vi "AllocateNewError.vi"(8 "ErrorIn":errorcluster, 10 "ErrorCode":i32, 11 "ConnectionIn":refnum<class "Connection.lvclass">) -> (0 "ErrorOut":errorcluster, 3 "ConnectionOut":refnum<class "Connection.lvclass">)   [LabVIEW 2021, in "ErrorDefinitionSQLite.lvclass"]
uses:
  ErrorDefinitionSQLite.lvclass
  ErrorDefinitionSQLite.lvclass/ErrorDefinitionSQLite.ctl
  <vilib>/drjdpowell/SQLite Library/SQLite.lvlib
  <vilib>/drjdpowell/SQLite Library/SQL Connection/Execute SQL.vi
  <vilib>/drjdpowell/SQLite Library/SQL Connection/Connection.lvclass
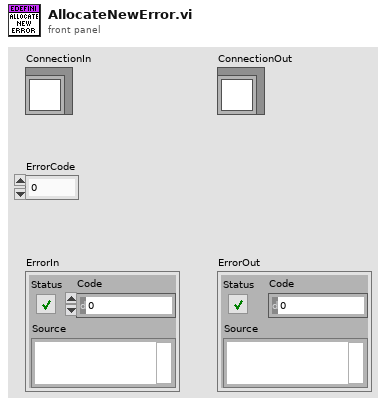
[diagram p1: front panel]
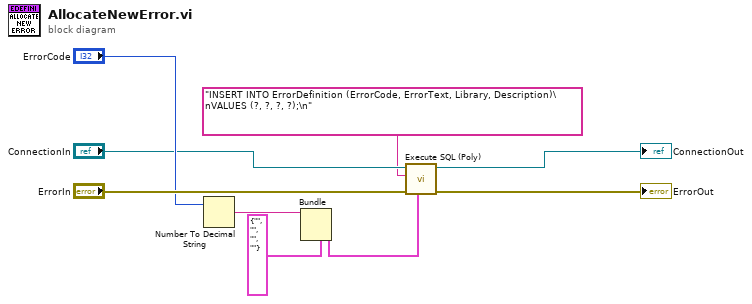
[diagram p0: block diagram]
diagram:
  n1 = Number To Decimal String(number="ErrorCode") -> (decimal integer string=w5:string)  [unwired: 1 in]
  n2 = Bundle(cluster=cluster{string, string, string, string} {"", "", "", ""}, w5) -> (w4:cluster{string, string, string, string})  [unwired: 3 in]
  n3 = call-poly <vilib>:"Execute SQL (Poly).vi"("Parameter(s)"=w4, "error in (no error)"="ErrorIn", "SQL"="INSERT INTO ErrorDefinition (ErrorCode, ErrorText, Library, Description)\nVALUES (?, ?, ?, ?);\n", "SQLite Connection in"="ConnectionIn") -> ("error out"=→"ErrorOut":errorcluster, "SQLite Connection"=→"ConnectionOut":refnum<class "Connection.lvclass">)  [unwired: 4 in, 2 out]
